vi "LCB Set Comm State.vi"(8 "error in (no error)":errorcluster caption="Fehler (Eingang, kein Fehler)", 11 "Device Handle":i64) -> (0 "error out":errorcluster caption="Fehler (Ausgang)")   [LabVIEW 2021, in "labbCAN_Bus_API.lvlib"]
doc: "LCB_Func long __stdcall LCB_SetCommState(dev_hdl hDev_in,\n unsigned char CommState);"
uses:
  labbCAN_Bus_API.lvlib
  CommState.ctl
  labbCAN_Bus_API.dll
panel:
  in  "Comm State":T1 items=["STOPPED"=2, "CONFIGURABLE"=128, "OPERATIONAL"=1]
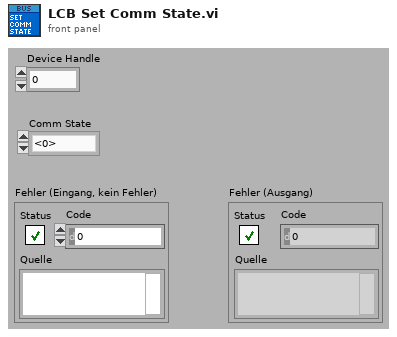
[diagram p1: front panel]
types:
  T1 = typedef "labbCAN_Bus_API.lvlib/CommState.ctl" = u8
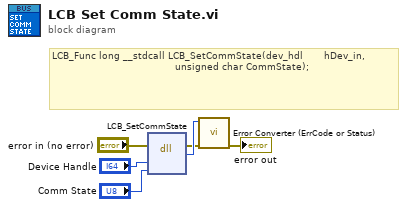
[diagram p0: block diagram]
diagram:
  # "LCB_Func long __stdcall LCB_SetCommState(dev_hdl       hDev_in,\n                                         unsigned char CommState);"
  n1 = dll-call lib="C:/Users/olaja/AppData/Local/CETONI_SDK/labbCAN_Bus_API.*" fn="LCB_SetCommState"(error in="error in (no error)", "hDev_in"="Device Handle", "CommState"="Comm State") -> (error out=w3:errorcluster, "Rückgabetyp"=w4:i32)  [unwired: 4 in, 1 out]
  n2 = call "Error Converter (ErrCode or Status).vi"("error in (no error)"=w3, "error code"=w4) -> ("error out"=→"error out":errorcluster)  [unwired: 9 in]
